vi "angle.vi"(9 "mic3":dbl, 10 "mic2":dbl, 11 "mic1":dbl) -> (3 "angle":dbl)   [LabVIEW 2014]
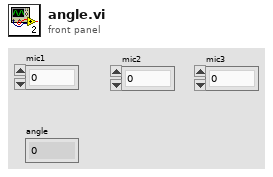
[diagram p1: front panel]
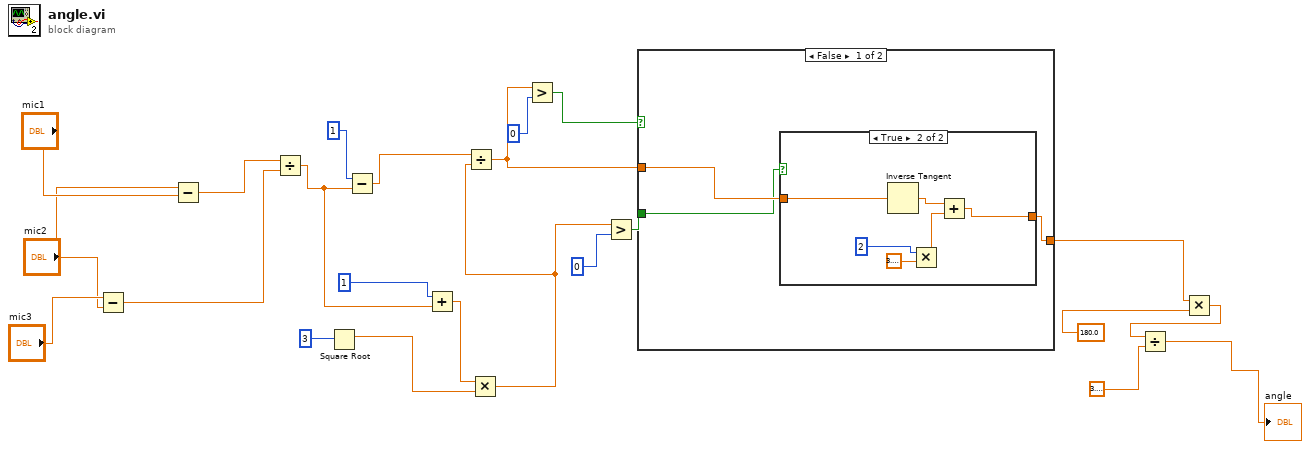
[diagram p0: block diagram]
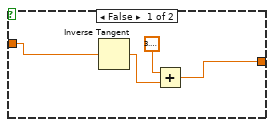
[diagram p2: hidden frame]
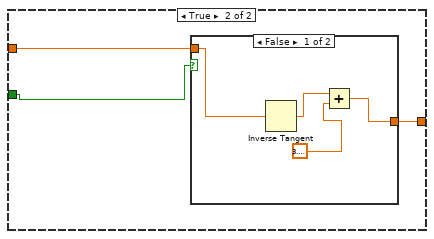
[diagram p3: hidden frame]
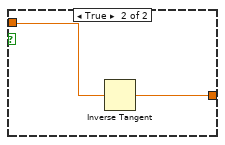
[diagram p4: hidden frame]
diagram:
  n1 = Subtract(x="mic3", y="mic2") -> (x-y=w18:dbl)
  n2 = Subtract(x="mic2", y="mic1") -> (x-y=w19:dbl)
  n3 = Divide(x=w19, y=w18) -> (x/y=w15:dbl)
  n4 = Square Root(x=3) -> (sqrt(x)=w4:dbl)
  n5 = Subtract(x=1, y=w15) -> (x-y=w10:dbl)
  n6 = Add(x=1, y=w15) -> (x+y=w14:dbl)
  n7 = Multiply(x=w14, y=w4) -> (x*y=w2:dbl)
  n8 = Divide(x=w10, y=w2) -> (x/y=w6:dbl)
  n9 = Greater?(x=w6, y=0) -> (0:w7:bool)
  n10 = Greater?(x=w2, y=0) -> (0:w1:bool)
  n11 = case shown="False" w7 {
    tunnel: w6 -> [w26 w39]
    tunnel: [w25 w38] -> w5
    tunnel: w1 -> [w24 w37]
    frame False {
      n12 = case shown="True" w24 {
        tunnel: w26 -> [w30 w36]
        tunnel: [w27 w34] -> w25
        frame False {
          n13 = Inverse Tangent(1:w30) -> (0:w29:dbl)
          n14 = Add(x=3.141592653589793, y=w29) -> (x+y=w27:dbl)
        }
        frame True {
          n15 = Inverse Tangent(1:w36) -> (0:w35:dbl)
          n16 = Multiply(x=2, y=3.141592653589793) -> (x*y=w31:dbl)
          n17 = Add(x=w35, y=w31) -> (x+y=w34:dbl)
        }
      }
    }
    frame True {
      n18 = case shown="False" w37 {
        tunnel: w39 -> [w43 w45]
        tunnel: [w40 w44] -> w38
        frame False {
          n19 = Inverse Tangent(1:w43) -> (0:w42:dbl)
          n20 = Add(x=w42, y=3.141592653589793) -> (x+y=w40:dbl)
        }
        frame True {
          n21 = Inverse Tangent(1:w45) -> (0:w44:dbl)
        }
      }
    }
  }
  n22 = Multiply(x=w5, y=180.0) -> (x*y=w12:dbl)
  n23 = Divide(x=w12, y=3.141592653589793) -> (x/y=→"angle":dbl)
